vi "getDataKinect.vi"(8 "Error In":errorcluster, 10 "Image 2":T3, 11 "KinectSensor References in":T1) -> (0 "Error Out":errorcluster, 1 "Image":T3(plugin-control), 2 "Joint Position":T2, 3 "KinectSensor References":T1, 4 "Boolean":bool)   [LabVIEW 2013]
uses:
  <vilib>/MakerHub/KinectOne/Private/Type Defs/KinectSensor References.ctl
  Microsoft.Kinect
  C:/Program Files (x86)/National Instruments/LabVIEW 2013/vi.lib/MakerHub/KinectOne/Private/Libs/BodyFrameDataInterface.dll
  Program Files (x86)/National Instruments/LabVIEW 2013/vi.lib/MakerHub/KinectOne/Private/Libs/BodyFrameDataInterface.dll
  <vilib>/vision/Image Controls.llb/IMAQ Image.ctl
  <vilib>/MakerHub/KinectOne/Private/Type Defs/Joint Position.ctl
  <vilib>/MakerHub/KinectOne/Private/Type Defs/JointType.ctl
  <vilib>/MakerHub/KinectOne/Private/kinectRead [ColorFrame].vi
  <vilib>/MakerHub/KinectOne/Private/kinectRead [BodyFrame].vi
  <vilib>/MakerHub/KinectOne/KinectOne.lvlib
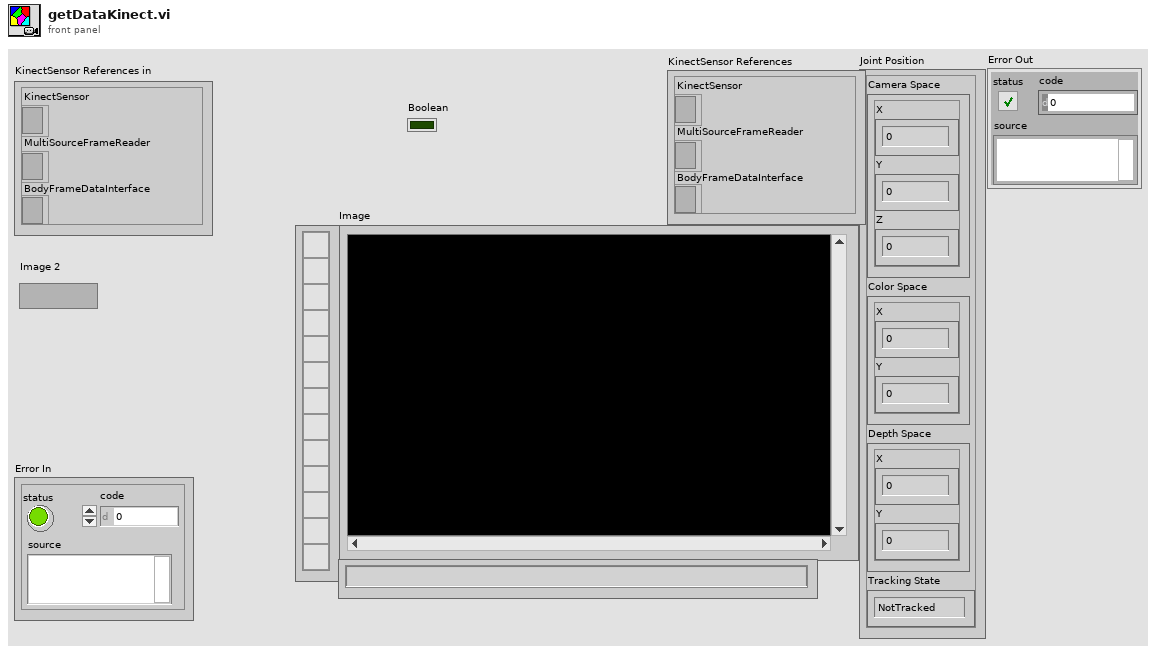
[diagram p1: front panel]
types:
  T1 = typedef "KinectOne.lvlib/KinectSensor References.ctl" = cluster{"KinectSensor":refnum<k24>, "MultiSourceFrameReader":refnum<k24>, "BodyFrameDataInterface":refnum<k24>}
  T2 = typedef "KinectOne.lvlib/Joint Position.ctl" = cluster{"Camera Space":cluster{"X":dbl, "Y":dbl, "Z":dbl}, "Color Space":cluster{"X":dbl, "Y":dbl}, "Depth Space":cluster{"X":dbl, "Y":dbl}, "Tracking State":enum16{"NotTracked", "Inferred", "Tracked"}}
  T3 = typedef "IMAQ Image.ctl" = refnum<image>
  T4 = typedef "KinectOne.lvlib/BodyData.ctl" = cluster{"ClippedEdges":T5, "HandLeftConfidence":T6, "HandLeftState":T7, "HandRightConfidence":T8, "HandRightState":T9, "IsRestricted":bool, "IsTracked":bool, "JointOrientations":refnum<k24>, "Joints":refnum<k24>, "Lean":refnum<k24>, "LeanTrackingState":T10, "TrackingId":u64}
  T5 = typedef "KinectOne.lvlib/ClippedEdges.ctl" = enum16{"None", "Right", "Left", "Top", "Bottom"}
  T6 = typedef "KinectOne.lvlib/HandLeftConfidence.ctl" = enum16{"Low", "High"}
  T7 = typedef "KinectOne.lvlib/HandLeftState.ctl" = enum16{"Unknown", "NotTracked", "Open", "Closed", "Lasso"}
  T8 = typedef "KinectOne.lvlib/HandRightConfidence.ctl" = enum16{"Low", "High"}
  T9 = typedef "KinectOne.lvlib/HandRightState.ctl" = enum16{"Unknown", "NotTracked", "Open", "Closed", "Lasso"}
  T10 = typedef "KinectOne.lvlib/LeanTrackingState.ctl" = enum16{"NotTracked", "Inferred", "Tracked"}
  T11 = typedef "KinectOne.lvlib/JointType.ctl" = enum16{"SpineBase", "SpineMid", "Neck", "Head", "ShoulderLeft", "ElbowLeft", "WristLeft", "HandLeft", "ShoulderRight", "ElbowRight", "WristRight", "HandRight", "HipLeft", "KneeLeft", "AnkleLeft", "FootLeft", "HipRight", "KneeRight", "AnkleRight", "FootRight", "SpineShoulder", "HandTipLeft", "ThumbLeft", "HandTipRight", "ThumbRight"}
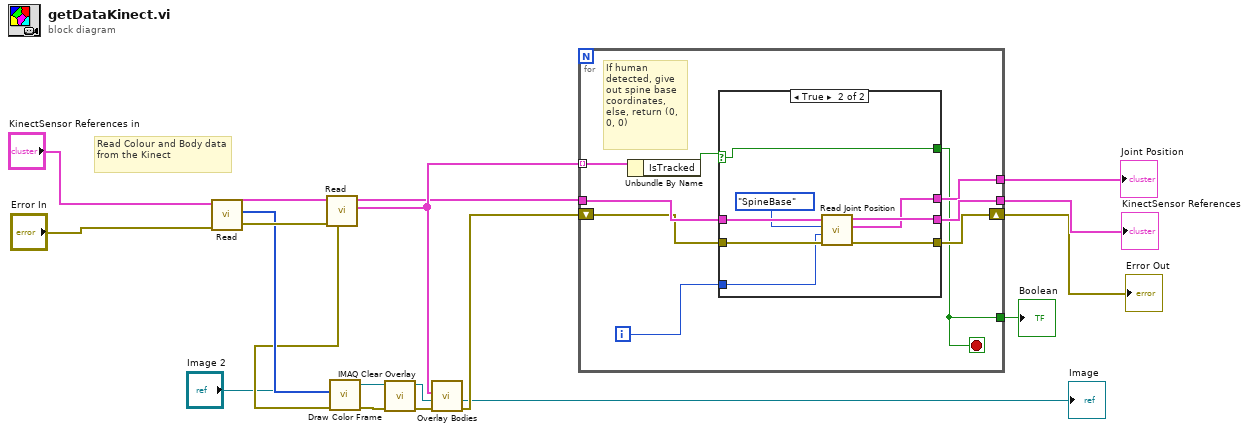
[diagram p0: block diagram]
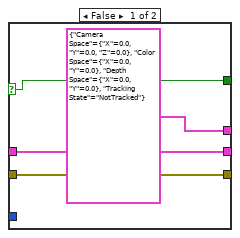
[diagram p2: hidden frame]
diagram:
  # "Read Colour and Body data from the Kinect"
  n1 = call-poly <vilib>:"Read.vi"("Error In"="Error In", "KinectSensor References in"="KinectSensor References in") -> ("Error Out"=w17:errorcluster, "frameData"=w12:u32[], "KinectSensor References out"=w16:T1)  [unwired: 7 in]
  n2 = call-poly <vilib>:"Read.vi"("error in (no error)"=w17, "KinectSensor References in"=w16) -> ("error out"=w11:errorcluster, "Body Data"=w19:T4[], "KinectSensor References out"=w18:T1)  [unwired: 7 in]
  n3 = call <vilib>:"Draw Color Frame.vi"("Error In"=w11, "U32 Array"=w12, "Image"="Image 2") -> ("Error Out"=w7:errorcluster, "Image Out"=w15:T3)  [unwired: 7 in]
  n4 = call "IMAQ Clear Overlay"("error in (no error)"=w7, "Image"=w15) -> ("error out"=w6:errorcluster, "Image Out"=w1:T3)  [unwired: 8 in]
  n5 = call <vilib>:"Overlay Bodies.vi"("Error In"=w6, "Image"=w1, "Body Data"=w19) -> ("Error Out"=w10:errorcluster, "Image Out"=→"Image":T3)  [unwired: 7 in]
  n6 = for {
    shift-right: [w23] -> w3
    shift-left: w10 -> [w24]
    tunnel: w19 -> [w28] mode=indexing
    tunnel: w18 -> [w27]
    tunnel: [w26] -> w4
    tunnel: [w25] -> w5
    tunnel: [w21] -> w2
    i -> [w20]
    stop <- w21 stop-if-true
    # "If human detected, give out spine base coordinates,\nelse, return (0, 0, 0)"
    n7 = Unbundle By Name(w28) -> ("IsTracked"=w22:bool)
    n8 = case shown="True" w22 {
      selector: w22 -> [w29 w36]
      tunnel: w27 -> [w32 w40]
      tunnel: [w32 w39] -> w26
      tunnel: [T2 {"Camera Space"={"X"=0.0, "Y"=0.0, "Z"=0.0}, "Color Space"={"X"=0.0, "Y"=0.0}, "Depth Space"={"X"=0.0, "Y"=0.0}, "Tracking State"=enum."NotTracked"} ("Joint Position") w37] -> w25
      tunnel: w24 -> [w30 w35]
      tunnel: [w30 w34] -> w23
      tunnel: [w29 w36] -> w21
      tunnel: w20 -> [_ w33]
      frame False {
      }
      frame True {
        n9 = call <vilib>:"Read Joint Position.vi"("Error In"=w35, "Body Index"=w33, "JointType"=JointType."SpineBase", "KinectSensor References"=w40) -> ("Error Out"=w34:errorcluster, "Joint Position"=w37:T2, "KinectSensor References"=w39:T1)  [unwired: 4 in, 1 out]
      }
    }
  }
  "Joint Position" <- w5
  "KinectSensor References" <- w4
  "Error Out" <- w3
  "Boolean" <- w2
